vi "Trapezoidal Waveform.vi"() -> ()   [LabVIEW 2019]
uses:
  <vilib>/Analysis/1siggen.llb/Ramp Pattern by Samples.vi
  <vilib>/Analysis/NI_AALBase.lvlib
panel:
  in  "Fase":dbl
  in  "Informação\nde amostragem":T1={"Amostras / s"=1000.0, "Quantidade\nde amostras"=1000.0} {"Amostras / s" format="%.2p"}
  in  "Amplitude":dbl
  out "Waveform Graph":waveform(dbl)(graph)
  in  "Frequencia":dbl
  in  "Offset":dbl
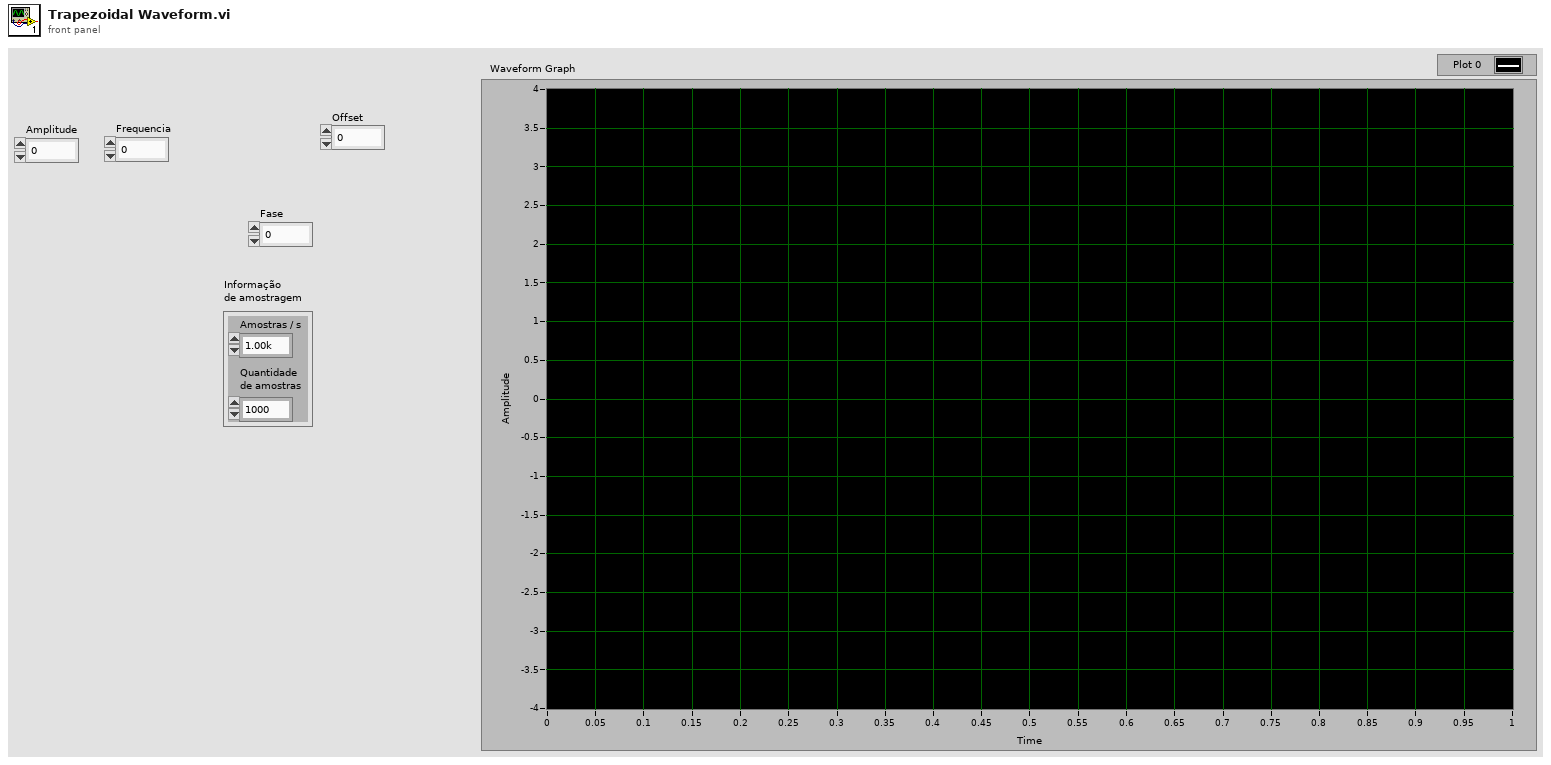
[diagram p1: front panel]
types:
  T1 = cluster{"Amostras / s":dbl, "Quantidade\nde amostras":dbl}
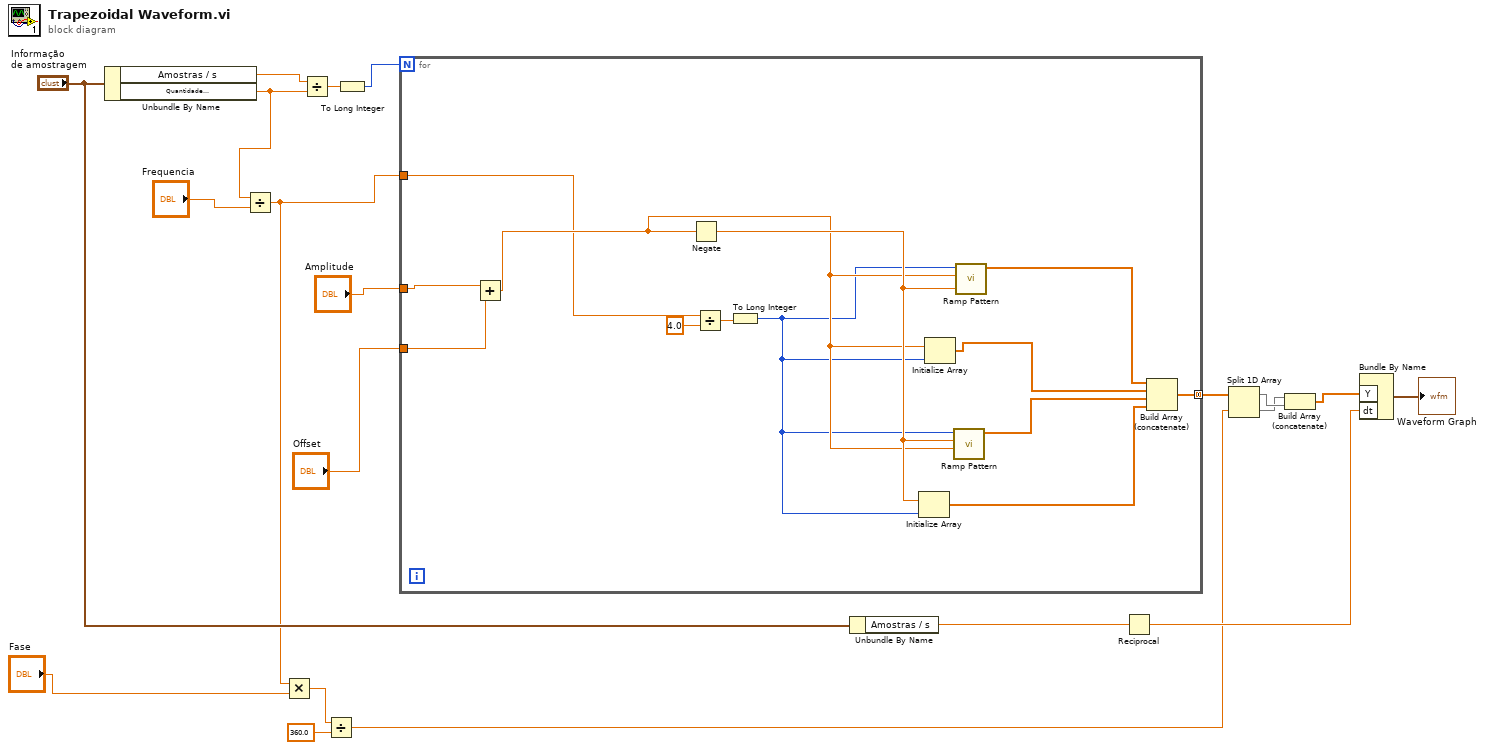
[diagram p0: block diagram]
diagram:
  n1 = Unbundle By Name("Informação\nde amostragem") -> ("Amostras / s"=w15:dbl, "Quantidade\nde amostras"=w11:dbl)
  n2 = Divide(x=w11, y="Frequencia") -> (x/y=w9:dbl)
  n3 = Multiply(x=w9, y="Fase") -> (x*y=w7:dbl)
  n4 = Divide(x=w15, y=w11) -> (x/y=w16:dbl)
  n5 = Divide(x=w7, y=360.0) -> (x/y=w4:dbl)
  n6 = To Long Integer(number=w16) -> (32bit integer=w14:i32)
  n7 = for {
    N: w14 -> [_]
    tunnel: "Amplitude" -> [w28]
    tunnel: [w29] -> w5 mode=concatenating
    tunnel: "Offset" -> [w27]
    tunnel: w9 -> [w21]
    n8 = Add(x=w28, y=w27) -> (x+y=w25:dbl)
    n9 = Negate(x=w25) -> (-x=w26:dbl)
    n10 = Divide(x=w21, y=4.0) -> (x/y=w23:dbl)
    n11 = To Long Integer(number=w23) -> (32bit integer=w22:i32)
    n12 = Initialize Array(w26, w22) -> (w30:dbl[])
    n13 = Initialize Array(w25, w22) -> (w31:dbl[])
    n14 = call-poly <vilib>:"Ramp Pattern.vi"("start"=w25, "end"=w26, "samples"=w22) -> ("Ramp Pattern"=w32:dbl[])  [unwired: 7 in, 1 out]
    n15 = call-poly <vilib>:"Ramp Pattern.vi"("start"=w26, "end"=w25, "samples"=w22) -> ("Ramp Pattern"=w33:dbl[])  [unwired: 7 in, 1 out]
    n16 = Build Array (concatenate)(w33, w31, w32, w30) -> (w29:dbl[])
  }
  n17 = Unbundle By Name("Informação\nde amostragem") -> ("Amostras / s"=w13:dbl)
  n18 = Reciprocal(x=w13) -> (1/x=w18:dbl)
  n19 = Split 1D Array(array=w5, index=w4) -> (first subarray=w3:dbl[], second subarray=w2:dbl[])
  n20 = Build Array (concatenate)(w2, w3) -> (w1:dbl[])
  n21 = Bundle By Name("Y"=w1, "dt"=w18) -> (→"Waveform Graph":waveform(dbl))  [unwired: 1 in]
